vi "Write Project to File.vi"(6 "Write":bool, 8 "error in":errorcluster, 11 "Project In":refnum<class "Project.lvclass">) -> (0 "error out":errorcluster, 2 "Continue?":bool, 3 "Project Out":refnum<class "Project.lvclass">)   [LabVIEW 2019, in "Panther Dashboard.lvlib" / "Project.lvclass"]
uses:
  Project.lvclass
  C:/GitClones/PantherDashboard/src/LabVIEW/Panther Dashboard/Class/LabVIEWItem/LabVIEWItem.lvclass
  LabVIEWItem/LabVIEWItem.lvclass/LabVIEWItem.ctl
  Project.lvclass/Project.ctl
  LabVIEWItem/Read Item Path.vi
  Read Target Name.vi
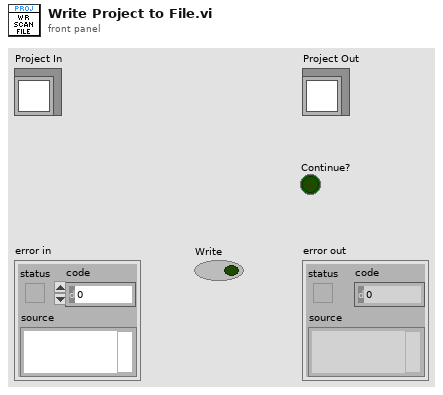
[diagram p1: front panel]
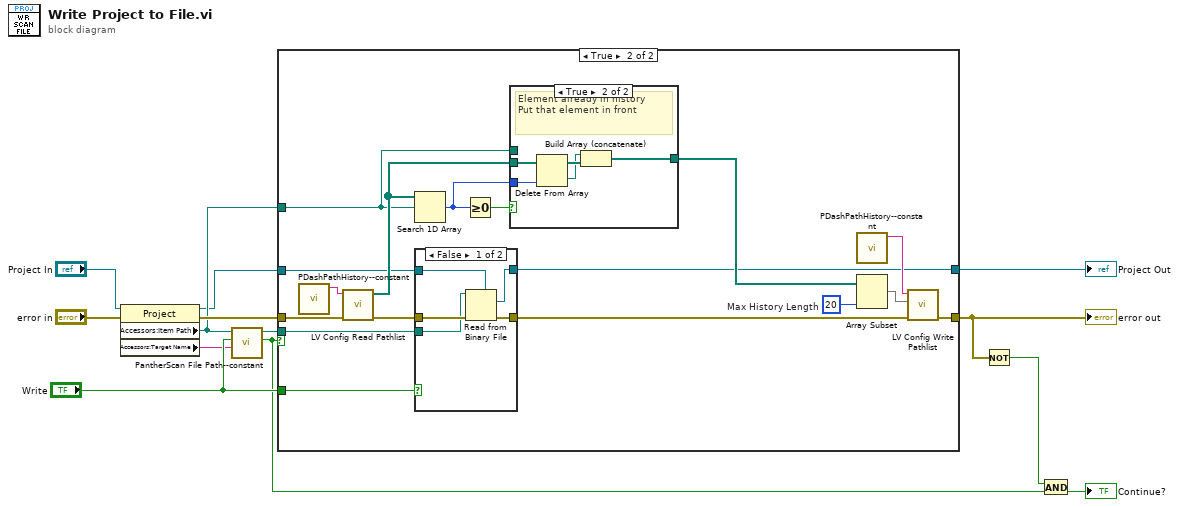
[diagram p0: block diagram]
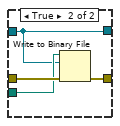
[diagram p3: hidden frame]
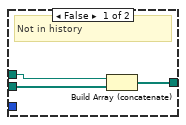
[diagram p4: hidden frame]
diagram:
  n1 = property class="Project"(reference="Project In", error in="error in") -> (reference out=w5:refnum<class "Project.lvclass">, error out=w12:errorcluster, "Accessors:Item Path"=w8:path, "Accessors:Target Name"=w7:string)
  n2 = call "PantherScan File Path--constant.vi"("Target"=w7, "Write"="Write", "Path"=w8) -> ("Continue?"=w9:bool, "PantherScan file Path"=w11:path)  [unwired: 7 in]
  n3 = case shown="True" w9 {
    tunnel: [w15 w32] -> w3
    tunnel: w12 -> [w15 w31]
    tunnel: w11 -> [_ w25]
    tunnel: w8 -> [_ w21]
    tunnel: [w14 w18] -> w4
    tunnel: "Write" -> [_ w17]
    tunnel: w5 -> [w14 w16]
    frame False {
      # "Scan Not Found, can't continue, call the init screen"
    }
    frame True {
      w22 = 20  # Max History Length
      n4 = call "PDashPathHistory--constant.vi"() -> ("PDashPathHistory"=w28:string)  [unwired: 11 in]
      n5 = call <resource>:"LV Config Read Pathlist.vi"("error in"=w31, "key"=w28) -> ("error out"=w30:errorcluster, "value"=w27:path[])  [unwired: 3 in, 1 out]
      n6 = Search 1D Array(1D array=w27, element=w21) -> (index of element=w19:i32)  [unwired: 1 in]
      n7 = case shown="False" w17 {
        tunnel: w30 -> [w37 w41]
        tunnel: [w36 w40] -> w29
        tunnel: w25 -> [w34 w39]
        tunnel: [w35 w38] -> w18
        tunnel: w16 -> [w33 w38]
        frame False {
          n8 = Read from Binary File(5:w33, 8:w37, 11:w34) -> (0:w36:errorcluster, 2:w35:refnum<class "Project.lvclass">)  [unwired: 3 in, 2 out]
        }
        frame True {
          n9 = Write to Binary File(file (use dialog)=w39, data=w38, error in=w41) -> (error out=w40:errorcluster)  [unwired: 3 in, 2 out]
        }
      }
      n10 = Greater Or Equal To 0?(x=w19) -> (x >= 0?=w26:bool)
      n11 = case shown="True" w26 {
        tunnel: w27 -> [w44 w49]
        tunnel: [w42 w47] -> w24
        tunnel: w21 -> [w43 _]
        tunnel: w19 -> [_ w48]
        frame False {
          # "Not in history"
          n12 = Build Array (concatenate)(w43, w44) -> (w42:path[])
        }
        frame True {
          # "Element already in history\nPut that element in front"
          n13 = Delete From Array(array=w49, index=w48) -> (deleted portion=w45:path, array with subset deleted=w46:path[])  [unwired: 1 in]
          n14 = Build Array (concatenate)(w45, w46) -> (w47:path[])
        }
      }
      n15 = call "PDashPathHistory--constant.vi"() -> ("PDashPathHistory"=w20:string)  [unwired: 11 in]
      n16 = Array Subset(array=w24, length=w22) -> (w23:path[])  [unwired: 1 in]
      n17 = call <resource>:"LV Config Write Pathlist.vi"("error in (no error)"=w29, "value"=w23, "key"=w20) -> ("error out"=w32:errorcluster)  [unwired: 4 in]
    }
  }
  "error out" <- w3
  "Project Out" <- w4
  n18 = Not(x=w3) -> (.not. x?=w1:bool)
  n19 = And(x=w1, y=w9) -> (x .and. y?=→"Continue?":bool)
